vi "Retrieve from DataBase.vi"(8 "error in (no error)":errorcluster, 10 "Search Criteria":string, 11 "Product DAO JSON in":refnum<class "Object DAO JSON.lvclass">) -> (0 "error out":errorcluster, 3 "Product DAO JSON out":refnum<class "Object DAO JSON.lvclass">)   [LabVIEW 2020, in "Object DAO JSON.lvclass"]
uses:
  Object DAO JSON.lvclass
  C:/Users/fflores/Desktop/DataBase - Copy - Copy - Copy/Object DAO/Object DAO.lvclass
  Object DAO JSON.lvclass/Object DAO JSON.ctl
  Object DAO/Object DAO.lvclass/Object DAO.ctl
  Object DAO/Member Accessors/Get Object Information.vi
  Object DAO/Member Accessors/Set Retrieved Items.vi
  <vilib>/JDP Science/JSONtext/JSONtext.lvlib
  External Libraries/JSON File Manipulation.lvlibp
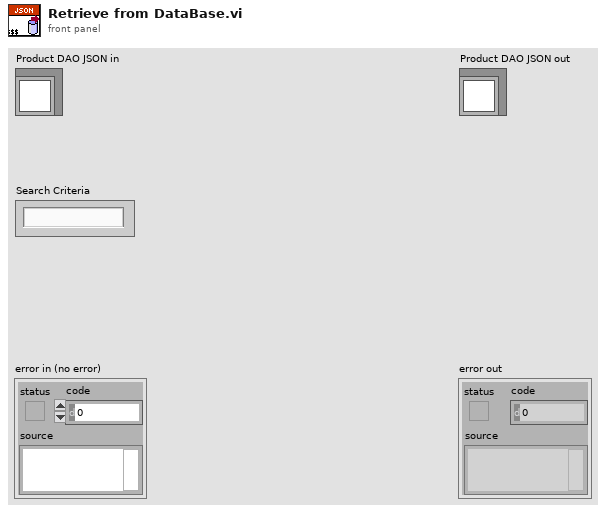
[diagram p1: front panel]
types:
  T1 = typedef "Object DAO.lvclass/Object Information.ctl" = cluster{"String":string, "Boolean":bool, "Numeric":dbl, "id":string}
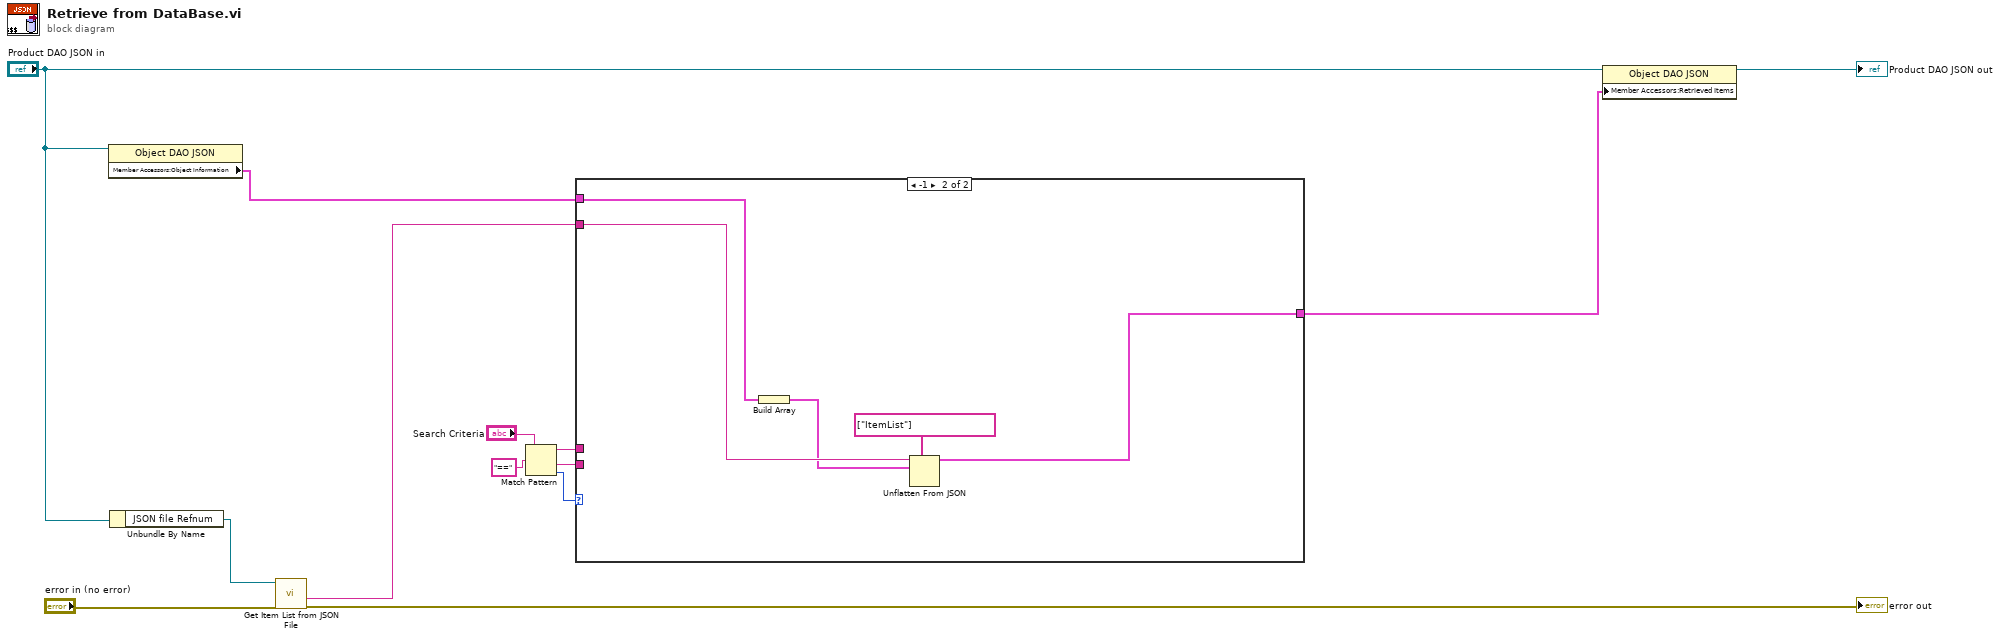
[diagram p0: block diagram]
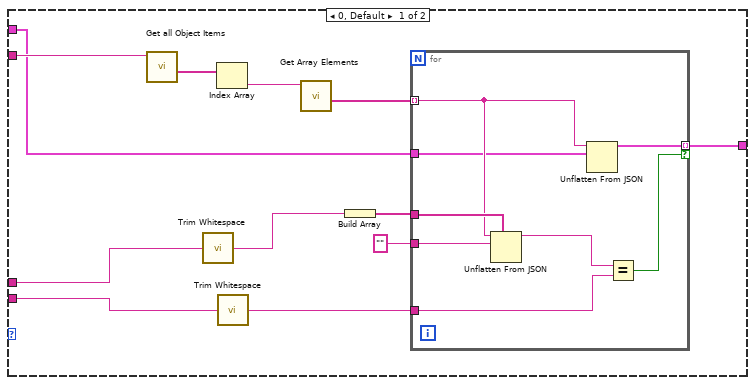
[diagram p2: hidden frame]
diagram:
  n1 = property class="Object DAO JSON"(reference="Product DAO JSON in") -> ("Member Accessors:Object Information"=w3:T1)  [unwired: 1 in, 2 out]
  n2 = Unbundle By Name("Product DAO JSON in") -> ("JSON file Refnum"=w13:refnum<file>)
  n3 = call "Get Item List from JSON File.vi"("error in (no error)"="error in (no error)", "Byte Stream File in"=w13) -> ("error out"=→"error out":errorcluster, "JSON String"=w4:string)  [unwired: 6 in, 2 out]
  n4 = Match Pattern(string="Search Criteria", regular expression="==") -> (before substring=w8:string, after substring=w7:string, offset past match=w5:i32)  [unwired: 1 in, 1 out]
  n5 = case shown="-1" w5 {
    tunnel: w4 -> [w18 w38]
    tunnel: w3 -> [w17 w35]
    tunnel: [w14 w34] -> w1
    tunnel: w8 -> [w16 _]
    tunnel: w7 -> [w15 _]
    frame 0, Default {
      n6 = call <vilib>:"Get all Object Items.vi"("JSON"=w18) -> ("<JSON>"=w25:string[])  [unwired: 7 in, 3 out]
      n7 = call <vilib>:"Trim Whitespace.vi"("string"=w16) -> ("trimmed string"=w22:string)  [unwired: 1 in]
      n8 = Index Array(array=w25) -> (element=w24:string)  [unwired: 1 in]
      n9 = call <vilib>:"Trim Whitespace.vi"("string"=w15) -> ("trimmed string"=w19:string)  [unwired: 1 in]
      n10 = call <vilib>:"Get Array Elements.vi"("JSON"=w24) -> ("<JSON>"=w23:string[])  [unwired: 8 in, 2 out]
      n11 = Build Array(w22) -> (w21:string[])
      n12 = for {
        tunnel: w23 -> [w29] mode=indexing
        tunnel: w21 -> [w33]
        tunnel: "" -> [w32]
        tunnel: w19 -> [w30]
        tunnel: w17 -> [w28]
        tunnel: [w27] -> w14 mode=indexing if=w26
        n13 = Unflatten From JSON(path=w33, JSON string=w29, type and defaults=w32) -> (value=w31:string)  [unwired: 4 in, 1 out]
        n14 = Unflatten From JSON(JSON string=w29, type and defaults=w28) -> (value=w27:T1)  [unwired: 5 in, 1 out]
        n15 = Equal?(x=w31, y=w30) -> (x = y?=w26:bool)
      }
    }
    frame -1 {
      n16 = Build Array(w35) -> (w36:T1[])
      n17 = Unflatten From JSON(path=string[] ["ItemList"], JSON string=w38, type and defaults=w36) -> (value=w34:T1[])  [unwired: 4 in, 1 out]
    }
  }
  n18 = property class="Object DAO JSON"(reference="Product DAO JSON in", "Member Accessors:Retrieved Items"=w1) -> (reference out=→"Product DAO JSON out":refnum<class "Object DAO JSON.lvclass">)  [unwired: 1 in, 1 out]
